vi "Get Group Configurations.vi"(8 "error in (no error)":errorcluster, 11 "Thread Configuration in":refnum<class "Thread Configuration.lvclass">) -> (0 "error out":errorcluster, 2 "Group Configurations":refnum<class "Group Configuration.lvclass">[](array[class]), 3 "Thread Configuration out":refnum<class "Thread Configuration.lvclass">)   [LabVIEW 2019, in "DSF Core.lvlib" / "Thread Configuration.lvclass"]
uses:
  Thread Configuration.lvclass
  Group/Group Configuration.lvclass
  Thread Configuration.lvclass/Thread Configuration.ctl
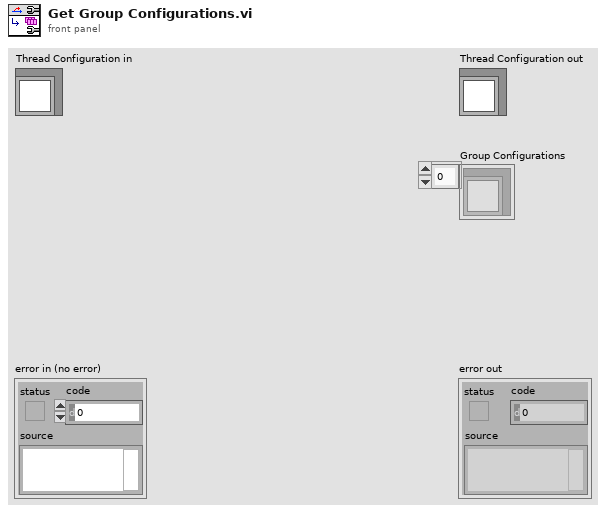
[diagram p1: front panel]
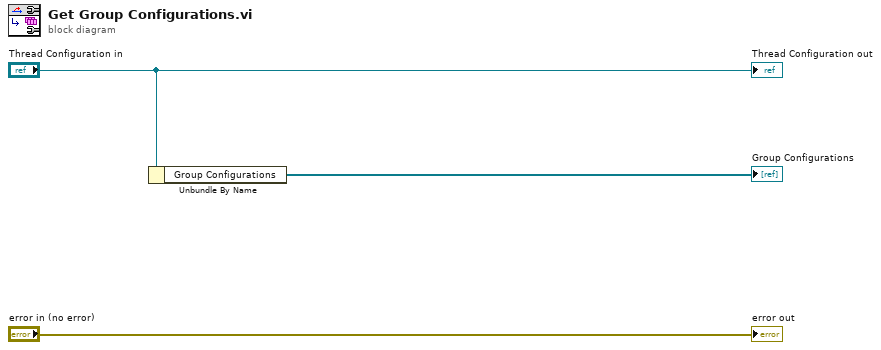
[diagram p0: block diagram]
diagram:
  n1 = Unbundle By Name("Thread Configuration in") -> ("Group Configurations"=→"Group Configurations":refnum<class "Group Configuration.lvclass">[])
  "error out" <- "error in (no error)"
  "Thread Configuration out" <- "Thread Configuration in"
